vi "Read CCD obj.vi"(8 "error in (no error)":errorcluster, 11 "CCD Configuration in":refnum<class "CCD Configuration.lvclass">) -> (0 "error out":errorcluster, 2 "Hardware.lvlib:CCD.lvlib:CCD.lvclass":refnum<class "CCD.lvclass">, 3 "CCD Configuration out":refnum<class "CCD Configuration.lvclass">)   [LabVIEW 2016, in "Hardware.lvlib" / "CCD.lvlib" / "CCD Configuration.lvclass"]
uses:
  <userlib>/Common Components/Hardware/CCD/CCD Configuration.lvclass
  <userlib>/Common Components/Hardware/CCD/CCD/CCD.lvclass
  <userlib>/Common Components/Hardware/CCD/CCD Configuration.lvclass/CCD Configuration.ctl
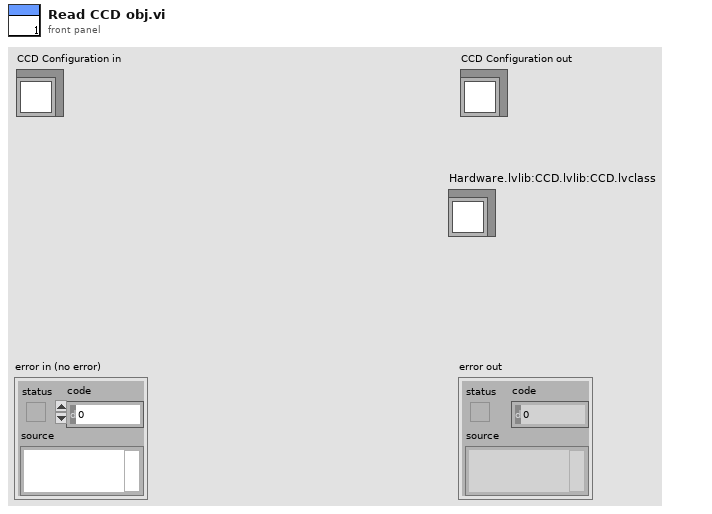
[diagram p1: front panel]
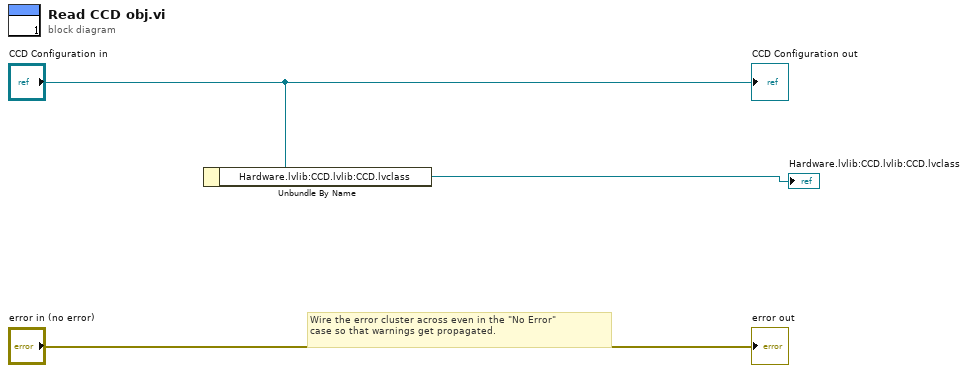
[diagram p0: block diagram]
diagram:
  # "Wire the error cluster across even in the \"No Error\"\ncase so that warnings get propagated."
  n1 = Unbundle By Name("CCD Configuration in") -> ("Hardware.lvlib:CCD.lvlib:CCD.lvclass"=→"Hardware.lvlib:CCD.lvlib:CCD.lvclass":refnum<class "CCD.lvclass">)
  "error out" <- "error in (no error)"
  "CCD Configuration out" <- "CCD Configuration in"
